vi "main.vi"() -> ()   [LabVIEW 2013]
uses:
  <vilib>/Utility/file.llb/Read From Spreadsheet File (DBL).vi
panel:
  out "Current file num":i32
  out "ROI Width":u32
  out "ROI Height":u32
  in  "Image Dark":dbl[][](array[numeric])
  in  "Image Light":dbl[][](array[numeric])
  in  "Image Atom":dbl[][](array[numeric])
  out "Best fit parameters":dbl[](array[numeric])
  out "Fitting Results Save Path":string[](array[string])
  out "Best fit results":dbl[][](array[numeric])
  in  "Initial guess values":dbl[](array[numeric])
  in  "Latest image data":dbl[][](array[numeric])
  out "Fitting Type":u16(ring)
  out "Force Guess?":bool
  out "Aquired?":bool
  out "Process Index":i32
  out "External Trigger":bool
  out "XY图":cluster{dbl[], dbl[]}[](graph)
  out "OD Image":dbl[][](graph)
  in  "OD fit":bool
  in  "OD num":i32
  out "Fit Done":bool
  in  "Exit":bool
  out "XY图 2":cluster{dbl[], dbl[]}[](graph)
  in  "Auto Split":bool
  in  "Fit":bool
  in  "Open File":bool
  in  "Auto Fit":bool
  in  "Stop":bool
  in  "Aquire":bool
  in  "Fitting Config":bool
  in  "Camera Config":bool
  in  "Initialize":bool
  in  "Live Image Display":refnum<k7>(container)
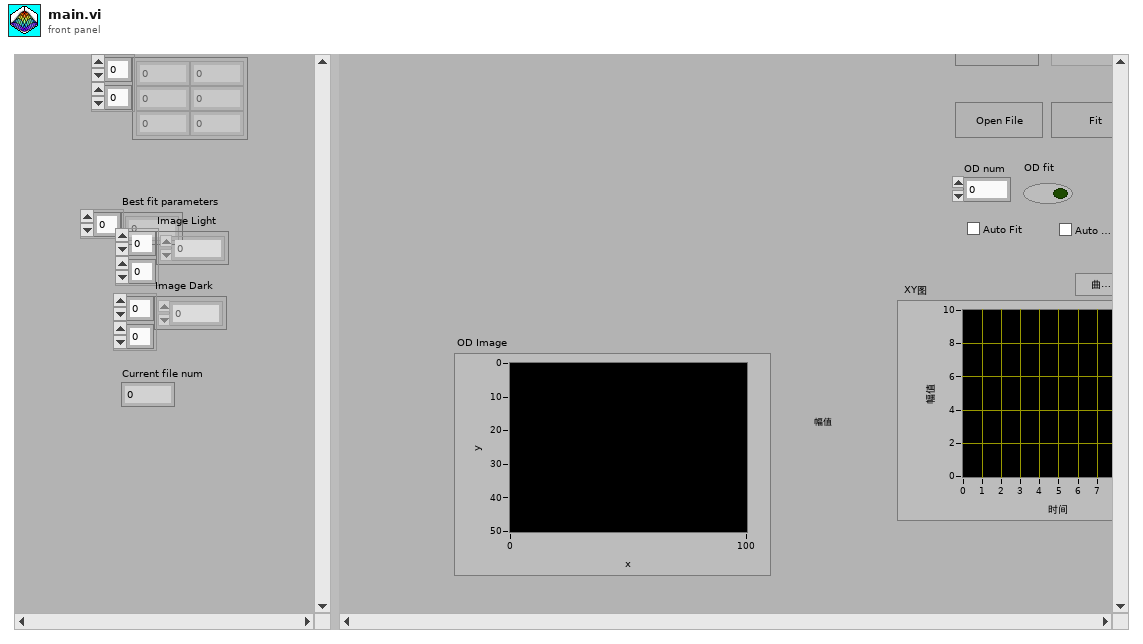
[diagram p1: front panel]
types:
  T1 = enum8{"Enabled", "Disabled", "Disabled and Grayed Out"}
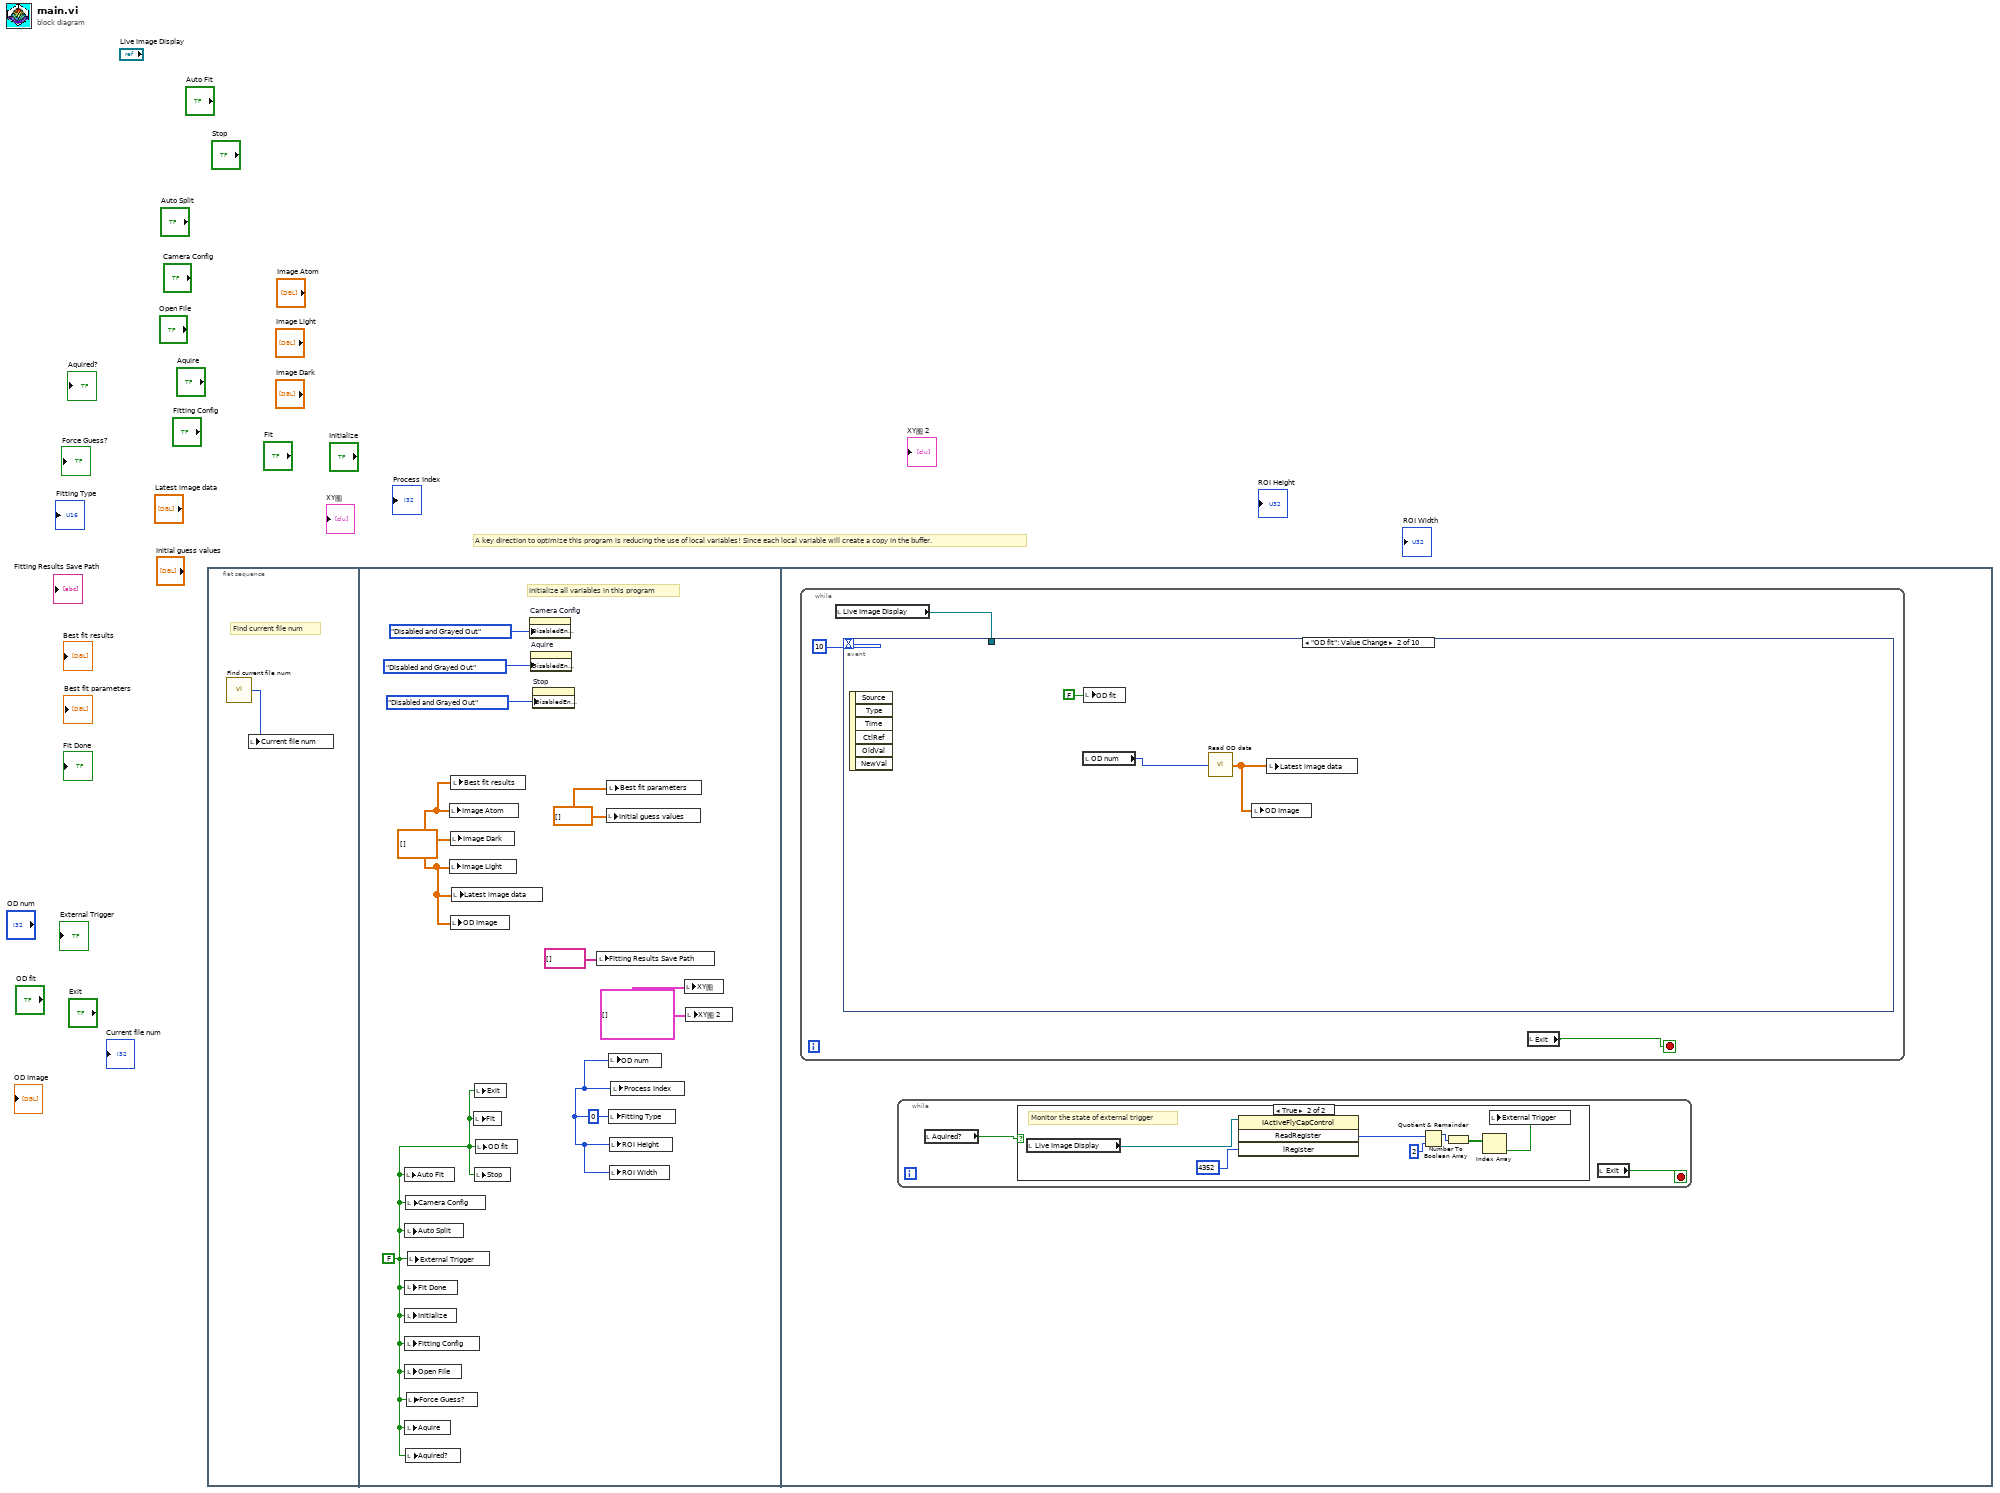
[diagram p0: block diagram]
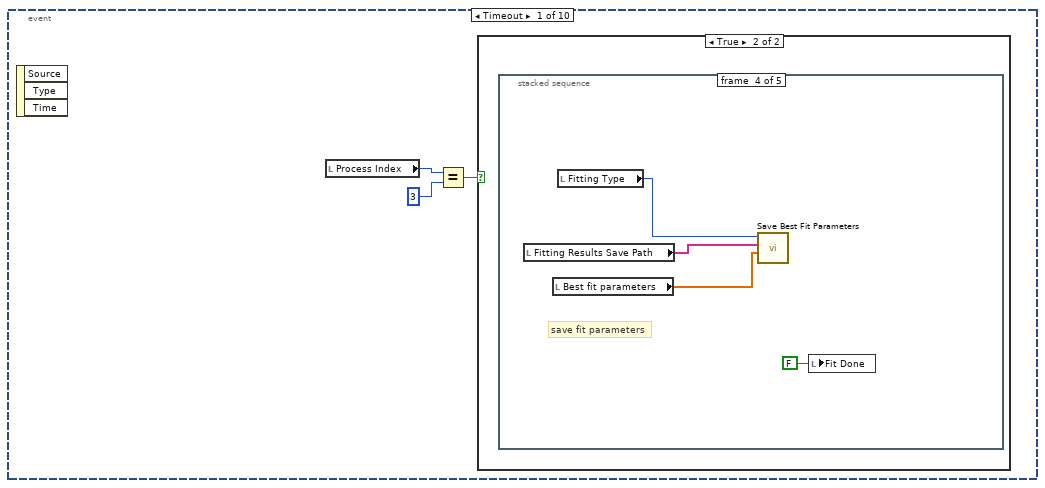
[diagram p3: hidden frame]
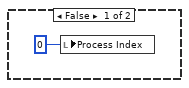
[diagram p4: hidden frame]
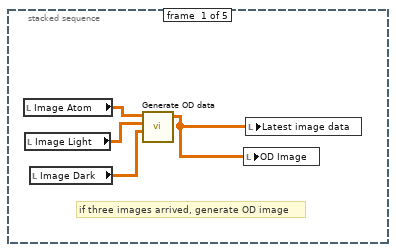
[diagram p5: hidden frame]
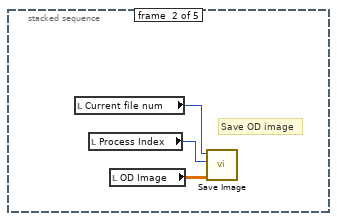
[diagram p6: hidden frame]
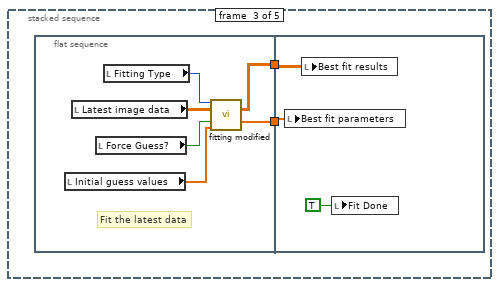
[diagram p7: hidden frame]
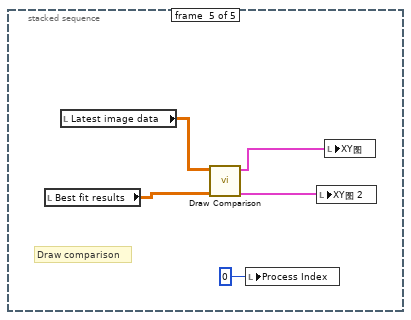
[diagram p8: hidden frame]
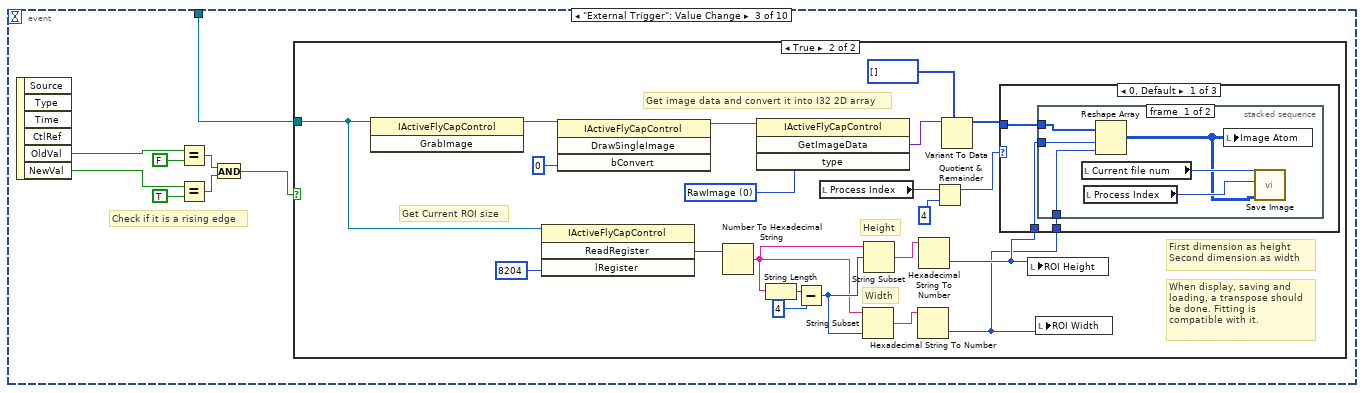
[diagram p9: hidden frame]
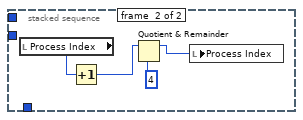
[diagram p11: hidden frame]
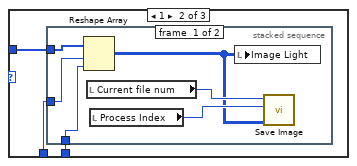
[diagram p12: hidden frame]
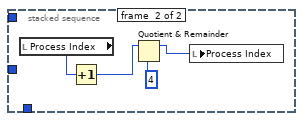
[diagram p13: hidden frame]
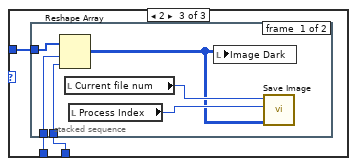
[diagram p14: hidden frame]
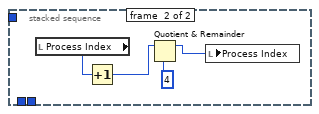
[diagram p15: hidden frame]
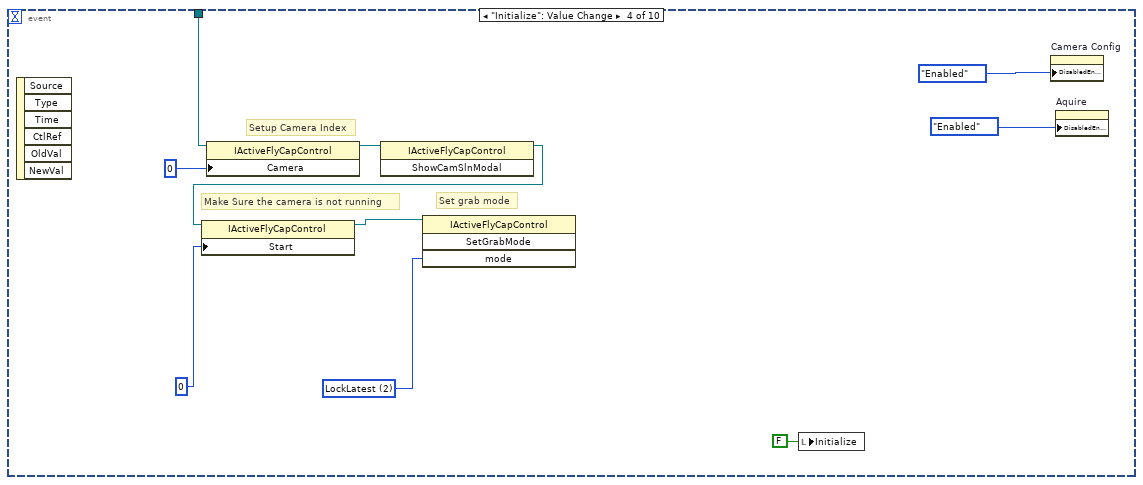
[diagram p16: hidden frame]
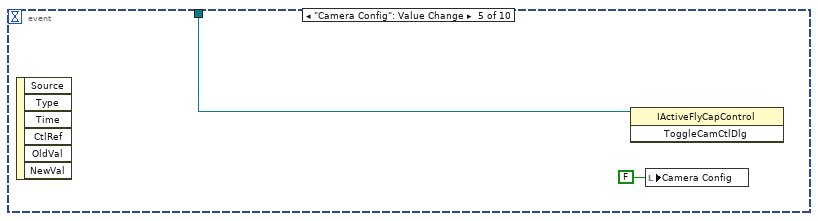
[diagram p17: hidden frame]
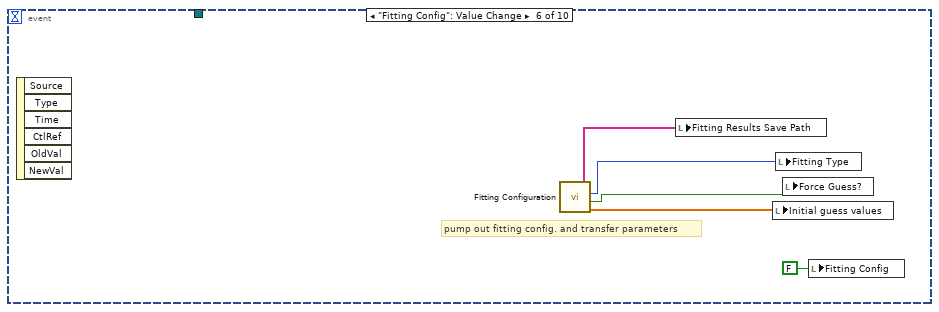
[diagram p18: hidden frame]
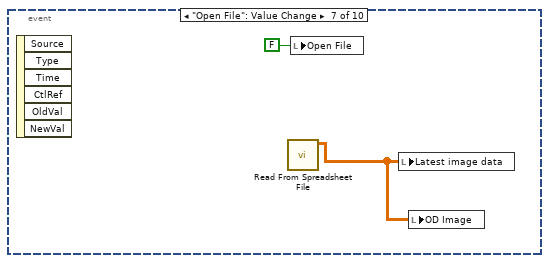
[diagram p19: hidden frame]
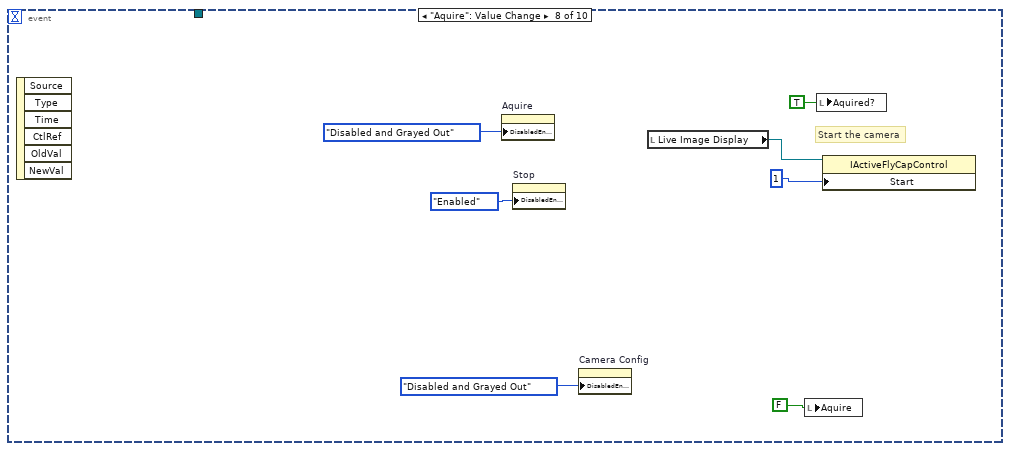
[diagram p20: hidden frame]
diagram:
  # "A key direction to optimize this program is reducing the use of local variables! Since each local variable will create a copy in the buffer."
  n1 = flat-sequence {
    frame #0 {
      # "Find current file num"
      n2 = call "Find current file num.vi"() -> ("Current File Num"=w1:u16)  [unwired: 2 in]
      n3 = local write "Current file num"(w1) -> ()
    }
    frame #1 {
      w4 = cluster{dbl[], dbl[]}[] [] ("XY图")
      w3 = 0 ("OD num")
      w7 = dbl[][] [] ("Best fit results")
      w6 = dbl[] [] ("Best fit parameters")
      w2 = FALSE ("Aquire")
      # "Initialize all variables in this program"
      n4 = local write "Auto Fit"(w2) -> ()
      n5 = local write "Auto Split"(w2) -> ()
      n6 = local write "Fit Done"(w2) -> ()
      n7 = local write "Initialize"(w2) -> ()
      n8 = local write "Fitting Config"(w2) -> ()
      n9 = local write "Open File"(w2) -> ()
      n10 = local write "Aquire"(w2) -> ()
      n11 = local write "Camera Config"(w2) -> ()
      n12 = local write "Aquired?"(w2) -> ()
      n13 = local write "Force Guess?"(w2) -> ()
      n14 = local write "External Trigger"(w2) -> ()
      n15 = local write "Image Atom"(w7) -> ()
      n16 = local write "Image Light"(w7) -> ()
      n17 = local write "Image Dark"(w7) -> ()
      n18 = local write "OD Image"(w7) -> ()
      n19 = local write "Best fit results"(w7) -> ()
      n20 = local write "Latest image data"(w7) -> ()
      n21 = local write "Fit"(w2) -> ()
      n22 = local write "Exit"(w2) -> ()
      n23 = local write "Stop"(w2) -> ()
      n24 = local write "OD fit"(w2) -> ()
      n25 = property on="Camera Config" class="Bool (strict)"("DisabledEnum"=T1."Disabled and Grayed Out" ("禁用")) -> ()  [unwired: 2 in, 2 out]
      n26 = property on="Aquire" class="Bool (strict)"("DisabledEnum"=T1."Disabled and Grayed Out" ("禁用")) -> ()  [unwired: 2 in, 2 out]
      n27 = property on="Stop" class="Bool (strict)"("DisabledEnum"=T1."Disabled and Grayed Out" ("禁用")) -> ()  [unwired: 2 in, 2 out]
      n28 = local write "Fitting Results Save Path"(string[] [] ("Fitting Results Save Path")) -> ()
      n29 = local write "Initial guess values"(w6) -> ()
      n30 = local write "Best fit parameters"(w6) -> ()
      n31 = local write "OD num"(w3) -> ()
      n32 = local write "Fitting Type"(w3) -> ()
      n33 = local write "ROI Height"(w3) -> ()
      n34 = local write "ROI Width"(w3) -> ()
      n35 = local write "Process Index"(w3) -> ()
      n36 = local write "XY图"(w4) -> ()
      n37 = local write "XY图 2"(w4) -> ()
    }
    frame #2 {
      n38 = while {
        stop <- w20 stop-if-true
        n39 = local read "Live Image Display"() -> (w21:refnum<k7>)
        n40 = event shown="[1] \"OD fit\": Value Change" {
          selector: _ -> [_ _ _ _ _ _ _ _ _ _]
          dyn-events: _ -> [_ _ _ _ _ _ _ _ _ _]
          timeout: 10 -> [_ _ _ _ _ _ _ _ _ _]
          tunnel: w21 -> [_ _ w57 w128 w136 _ _ _ _ _]
          event Timeout {
            n41 = event-data() -> ()  [unwired: 1 in, 3 out]
            n42 = local read "Process Index"() -> (w25:i32)
            n43 = Equal?(x=w25, y=3) -> (x = y?=w23:bool)
            n44 = case shown="True" w23 {
              frame False {
                n45 = local write "Process Index"(0 ("Process Index")) -> ()
              }
              frame True {
                n46 = stacked-sequence {
                  frame #0 {
                    # "if three images arrived, generate OD image"
                    n47 = local read "Image Atom"() -> (w30:dbl[][])
                    n48 = local read "Image Light"() -> (w29:dbl[][])
                    n49 = local read "Image Dark"() -> (w28:dbl[][])
                    n50 = call "Generate OD data.vi"("dark"=w28, "light"=w29, "atom"=w30) -> ("OD image"=w27:dbl[][])  [unwired: 3 in]
                    n51 = local write "OD Image"(w27) -> ()
                    n52 = local write "Latest image data"(w27) -> ()
                  }
                  frame #1 {
                    # "Save OD image"
                    n53 = local read "Current file num"() -> (w33:i32)
                    n54 = local read "Process Index"() -> (w32:i32)
                    n55 = local read "OD Image"() -> (w31:dbl[][])
                    n56 = call "Save Image.vi"("Data"=w31, "Process Index"=w32, "Current File Num"=w33) -> ()  [unwired: 9 in]
                  }
                  frame #2 {
                    n57 = flat-sequence {
                      tunnel: [w37] -> w35
                      tunnel: [w36] -> w34
                      tunnel: w35 -> [w44]
                      tunnel: w34 -> [w43]
                      frame #0 {
                        # "Fit the latest data"
                        n58 = local read "Initial guess values"() -> (w38:dbl[])
                        n59 = local read "Latest image data"() -> (w40:dbl[][])
                        n60 = local read "Force Guess?"() -> (w39:bool)
                        n61 = local read "Fitting Type"() -> (w41:u16)
                        n62 = call "fitting modified.vi"("fitting type"=w41, "2D data"=w40, "force guess?"=w39, "intial guess value"=w38) -> ("best fit"=w37:dbl[][], "best fit parameters"=w36:dbl[])  [unwired: 9 in, 1 out]
                      }
                      frame #1 {
                        n63 = local write "Best fit parameters"(w43) -> ()
                        n64 = local write "Best fit results"(w44) -> ()
                        n65 = local write "Fit Done"(TRUE ("Fit Done")) -> ()
                      }
                    }
                  }
                  frame #3 {
                    # "save fit parameters"
                    n66 = local read "Fitting Results Save Path"() -> (w47:string[])
                    n67 = local read "Best fit parameters"() -> (w46:dbl[])
                    n68 = local read "Fitting Type"() -> (w48:u16)
                    n69 = call "Save Best Fit Parameters.vi"("Best Fit Parameters"=w46, "Fitting Results Save Path"=w47, "Fitting Type"=w48) -> ()  [unwired: 9 in]
                    n70 = local write "Fit Done"(FALSE ("Fit Done")) -> ()
                  }
                  frame #4 {
                    # "Draw comparison"
                    n71 = local read "Best fit results"() -> (w51:dbl[][])
                    n72 = local read "Latest image data"() -> (w50:dbl[][])
                    n73 = call "Draw Comparison.vi"("Best Fit"=w51, "Raw Data"=w50) -> ("Vertical Comparison"=w52:cluster{i32[], dbl[]}[], "Horizontal Comparison"=w53:cluster{i32[], dbl[]}[])  [unwired: 7 in]
                    n74 = local write "Process Index"(0 ("Process Index")) -> ()
                    n75 = local write "XY图 2"(w52) -> ()
                    n76 = local write "XY图"(w53) -> ()
                  }
                }
              }
            }
          }
          event "OD fit": Value Change {
            n77 = event-data() -> ()  [unwired: 1 in, 6 out]
            n78 = local read "OD num"() -> (w55:i32)
            n79 = local write "OD fit"(FALSE ("OD fit")) -> ()
            n80 = call "Read OD data.vi"("OD num"=w55) -> ("OD data"=w54:dbl[][])  [unwired: 4 in]
            n81 = local write "OD Image"(w54) -> ()
            n82 = local write "Latest image data"(w54) -> ()
          }
          event "External Trigger": Value Change {
            # "Check if it is a rising edge"
            n83 = event-data() -> ("OldVal"=w62:bool, "NewVal"=w61:bool)  [unwired: 1 in, 4 out]
            n84 = Equal?(x=w62, y=FALSE) -> (x = y?=w64:bool)
            n85 = Equal?(x=w61, y=TRUE) -> (x = y?=w63:bool)
            n86 = And(x=w64, y=w63) -> (x .and. y?=w58:bool)
            n87 = case shown="True" w58 {
              tunnel: w57 -> [_ w81]
              frame False {
              }
              frame True {
                w82 = 0 items=["RawImage", "ColorProcessedImage"] ("type")
                # "Get image data and convert it into I32 2D array"
                # "When display, saving and \nloading, a transpose should\nbe done. Fitting is \ncompatible with it."
                # "First dimension as height\nSecond dimension as width"
                # "Width"
                # "Height"
                # "Get Current ROI size"
                n88 = invoke class="IActiveFlyCapControl" method="GrabImage"(reference=w81) -> (reference out=w85:refnum<k7>)  [unwired: 2 in, 2 out]
                n89 = invoke class="IActiveFlyCapControl" method="ReadRegister"(reference=w81, "lRegister"=u32 8204) -> ("ReadRegister"=w78:u32)  [unwired: 2 in, 3 out]
                n90 = invoke class="IActiveFlyCapControl" method="DrawSingleImage"(reference=w85, "bConvert"=0) -> (reference out=w84:refnum<k7>)  [unwired: 2 in, 3 out]
                n91 = Number To Hexadecimal String(2:w78) -> (0:w74:string)  [unwired: 1 in]
                n92 = invoke class="IActiveFlyCapControl" method="GetImageData"(reference=w84, "type"=w82) -> ("GetImageData"=w79:variant)  [unwired: 2 in, 3 out]
                n93 = String Length(string=w74) -> (length=w77:i32)
                n94 = Subtract(x=w77, y=4) -> (x-y=w75:i32)
                n95 = local read "Process Index"() -> (w70:i32)
                n96 = String Subset(string=w74, length (rest)=w75) -> (substring=w71:string)  [unwired: 1 in]
                n97 = String Subset(string=w74, offset (0)=w75) -> (substring=w72:string)  [unwired: 1 in]
                n98 = Hexadecimal String To Number(string=w71) -> (number=w65:u32)  [unwired: 2 in, 1 out]
                n99 = Hexadecimal String To Number(string=w72) -> (number=w66:u32)  [unwired: 2 in, 1 out]
                n100 = Quotient & Remainder(x=w70, y=4) -> (x-y*floor(x/y)=w68:i32)  [unwired: 1 out]
                n101 = Variant To Data(type=i32[] [], Variant=w79) -> (data=w67:i32[])  [unwired: 1 in, 1 out]
                n102 = case shown="0, Default" w68 {
                  tunnel: w67 -> [w88 w101 w114]
                  tunnel: w66 -> [w87 w100 w113]
                  tunnel: w65 -> [w86 w99 w112]
                  frame 0, Default {
                    n103 = stacked-sequence {
                      tunnel: w88 -> [w92 _]
                      tunnel: w87 -> [w91 _]
                      tunnel: w86 -> [w90 _]
                      frame #0 {
                        n104 = local read "Current file num"() -> (w94:i32)
                        n105 = local read "Process Index"() -> (w93:i32)
                        n106 = Reshape Array(w92, w91, w90) -> (w89:i32[][])
                        n107 = local write "Image Atom"(w89) -> ()
                        n108 = call "Save Image.vi"("Data"=w89, "Process Index"=w93, "Current File Num"=w94) -> ()  [unwired: 9 in]
                      }
                      frame #1 {
                        n109 = local read "Process Index"() -> (w98:i32)
                        n110 = Increment(x=w98) -> (x+1=w97:i32)
                        n111 = Quotient & Remainder(x=w97, y=4) -> (x-y*floor(x/y)=w95:i32)  [unwired: 1 out]
                        n112 = local write "Process Index"(w95) -> ()
                      }
                    }
                  }
                  frame 1 {
                    n113 = stacked-sequence {
                      tunnel: w101 -> [w103 _]
                      tunnel: w100 -> [w105 _]
                      tunnel: w99 -> [w104 _]
                      frame #0 {
                        n114 = Reshape Array(w103, w105, w104) -> (w102:i32[][])
                        n115 = local read "Current file num"() -> (w107:i32)
                        n116 = local read "Process Index"() -> (w106:i32)
                        n117 = local write "Image Light"(w102) -> ()
                        n118 = call "Save Image.vi"("Data"=w102, "Process Index"=w106, "Current File Num"=w107) -> ()  [unwired: 9 in]
                      }
                      frame #1 {
                        n119 = local read "Process Index"() -> (w111:i32)
                        n120 = Increment(x=w111) -> (x+1=w110:i32)
                        n121 = Quotient & Remainder(x=w110, y=4) -> (x-y*floor(x/y)=w108:i32)  [unwired: 1 out]
                        n122 = local write "Process Index"(w108) -> ()
                      }
                    }
                  }
                  frame 2 {
                    n123 = stacked-sequence {
                      tunnel: w114 -> [w118 _]
                      tunnel: w113 -> [w117 _]
                      tunnel: w112 -> [w116 _]
                      frame #0 {
                        n124 = Reshape Array(w118, w117, w116) -> (w115:i32[][])
                        n125 = local read "Current file num"() -> (w120:i32)
                        n126 = local read "Process Index"() -> (w119:i32)
                        n127 = local write "Image Dark"(w115) -> ()
                        n128 = call "Save Image.vi"("Data"=w115, "Process Index"=w119, "Current File Num"=w120) -> ()  [unwired: 9 in]
                      }
                      frame #1 {
                        n129 = local read "Process Index"() -> (w124:i32)
                        n130 = Increment(x=w124) -> (x+1=w123:i32)
                        n131 = Quotient & Remainder(x=w123, y=4) -> (x-y*floor(x/y)=w121:i32)  [unwired: 1 out]
                        n132 = local write "Process Index"(w121) -> ()
                      }
                    }
                  }
                }
                n133 = local write "ROI Height"(w66) -> ()
                n134 = local write "ROI Width"(w65) -> ()
              }
            }
          }
          event "Initialize": Value Change {
            w132 = 2 items=["FreeRunning", "LockNext", "LockLatest"] ("mode")
            # "Setup Camera Index"
            # "Set grab mode"
            # "Make Sure the camera is not running"
            n135 = event-data() -> ()  [unwired: 1 in, 6 out]
            n136 = property class="IActiveFlyCapControl"(reference=w128, "Camera"=0 ("Start")) -> (reference out=w131:refnum<k7>)  [unwired: 1 in, 1 out]
            n137 = invoke class="IActiveFlyCapControl" method="ShowCamSlnModal"(reference=w131) -> (reference out=w127:refnum<k7>)  [unwired: 2 in, 2 out]
            n138 = property class="IActiveFlyCapControl"(reference=w127, "Start"=0 ("Camera")) -> (reference out=w126:refnum<k7>)  [unwired: 1 in, 1 out]
            n139 = invoke class="IActiveFlyCapControl" method="SetGrabMode"(reference=w126, "mode"=w132) -> ()  [unwired: 2 in, 4 out]
            n140 = local write "Initialize"(FALSE ("Initialize")) -> ()
            n141 = property on="Camera Config" class="Bool (strict)"("DisabledEnum"=T1."Enabled" ("禁用")) -> ()  [unwired: 2 in, 2 out]
            n142 = property on="Aquire" class="Bool (strict)"("DisabledEnum"=T1."Enabled" ("禁用")) -> ()  [unwired: 2 in, 2 out]
          }
          event "Camera Config": Value Change {
            n143 = event-data() -> ()  [unwired: 1 in, 6 out]
            n144 = invoke class="IActiveFlyCapControl" method="ToggleCamCtlDlg"(reference=w136) -> ()  [unwired: 2 in, 3 out]
            n145 = local write "Camera Config"(FALSE ("Camera Config")) -> ()
          }
          event "Fitting Config": Value Change {
            # "pump out fitting config. and transfer parameters"
            n146 = event-data() -> ()  [unwired: 1 in, 6 out]
            n147 = call "Fitting Configuration.vi"() -> ("intial guess"=w140:dbl[], "Force Guess？"=w139:bool, "Fitting Type"=w138:u16, "Fitting Results Save Path"=w137:string[])  [unwired: 5 in]
            n148 = local write "Fitting Results Save Path"(w137) -> ()
            n149 = local write "Initial guess values"(w140) -> ()
            n150 = local write "Fitting Type"(w138) -> ()
            n151 = local write "Force Guess?"(w139) -> ()
            n152 = local write "Fitting Config"(FALSE ("Fitting Config")) -> ()
          }
          event "Open File": Value Change {
            n153 = event-data() -> ()  [unwired: 1 in, 6 out]
            n154 = call-poly <vilib>:"Read From Spreadsheet File.vi"() -> ("all rows"=w142:dbl[][])  [unwired: 7 in, 4 out]
            n155 = local write "Open File"(FALSE ("Open File")) -> ()
            n156 = local write "Latest image data"(w142) -> ()
            n157 = local write "OD Image"(w142) -> ()
          }
          event "Aquire": Value Change {
            # "Start the camera"
            n158 = event-data() -> ()  [unwired: 1 in, 6 out]
            n159 = property on="Aquire" class="Bool (strict)"("DisabledEnum"=T1."Disabled and Grayed Out" ("禁用")) -> ()  [unwired: 2 in, 2 out]
            n160 = property on="Stop" class="Bool (strict)"("DisabledEnum"=T1."Enabled" ("禁用")) -> ()  [unwired: 2 in, 2 out]
            n161 = property on="Camera Config" class="Bool (strict)"("DisabledEnum"=T1."Disabled and Grayed Out" ("禁用")) -> ()  [unwired: 2 in, 2 out]
            n162 = local read "Live Image Display"() -> (w145:refnum<k7>)
            n163 = local write "Aquire"(FALSE ("Initialize")) -> ()
            n164 = local write "Aquired?"(TRUE ("Aquired?")) -> ()
            n165 = property class="IActiveFlyCapControl"(reference=w145, "Start"=1) -> ()  [unwired: 1 in, 2 out]
          }
          event "Stop": Value Change {
            # "stop the camera"
            n166 = event-data() -> ()  [unwired: 1 in, 6 out]
            n167 = local read "Live Image Display"() -> (w153:refnum<k7>)
            n168 = local write "Stop"(FALSE ("Initialize")) -> ()
            n169 = property on="Stop" class="Bool (strict)"("DisabledEnum"=T1."Disabled and Grayed Out" ("禁用")) -> ()  [unwired: 2 in, 2 out]
            n170 = property on="Aquire" class="Bool (strict)"("DisabledEnum"=T1."Disabled and Grayed Out" ("禁用")) -> ()  [unwired: 2 in, 2 out]
            n171 = property class="IActiveFlyCapControl"(reference=w153, "Start"=0) -> (reference out=w152:refnum<k7>)  [unwired: 1 in, 1 out]
            n172 = local write "Aquired?"(FALSE ("Aquired?")) -> ()
            n173 = local write "Live Image Display"(w152) -> ()
          }
          event "Fit": Value Change {
            n174 = event-data() -> ()  [unwired: 1 in, 6 out]
            n175 = stacked-sequence {
              frame #0 {
                n176 = flat-sequence {
                  tunnel: [w161] -> w159
                  tunnel: [w160] -> w158
                  tunnel: w159 -> [w169]
                  tunnel: w158 -> [w168]
                  frame #0 {
                    # "Fit the latest data"
                    n177 = local read "Initial guess values"() -> (w164:dbl[])
                    n178 = local read "Latest image data"() -> (w163:dbl[][])
                    n179 = local read "Force Guess?"() -> (w165:bool)
                    n180 = local read "Fitting Type"() -> (w162:u16)
                    n181 = call "fitting modified.vi"("fitting type"=w162, "2D data"=w163, "force guess?"=w165, "intial guess value"=w164) -> ("best fit"=w161:dbl[][], "best fit parameters"=w160:dbl[])  [unwired: 9 in, 1 out]
                  }
                  frame #1 {
                    n182 = local write "Fit"(FALSE ("Fit")) -> ()
                    n183 = local write "Best fit results"(w169) -> ()
                    n184 = local write "Best fit parameters"(w168) -> ()
                    n185 = local write "Fit Done"(TRUE ("Fit Done")) -> ()
                  }
                }
              }
              frame #1 {
                # "Save best fit parameters"
                n186 = local read "Fitting Results Save Path"() -> (w171:string[])
                n187 = local read "Best fit parameters"() -> (w170:dbl[])
                n188 = local read "Fitting Type"() -> (w172:u16)
                n189 = call "Save Best Fit Parameters.vi"("Best Fit Parameters"=w170, "Fitting Results Save Path"=w171, "Fitting Type"=w172) -> ()  [unwired: 9 in]
                n190 = local write "Fit Done"(FALSE ("Fit Done")) -> ()
              }
              frame #2 {
                # "Draw Comparison"
                n191 = local read "Latest image data"() -> (w178:dbl[][])
                n192 = local read "Best fit results"() -> (w177:dbl[][])
                n193 = call "Draw Comparison.vi"("Best Fit"=w177, "Raw Data"=w178) -> ("Vertical Comparison"=w175:cluster{i32[], dbl[]}[], "Horizontal Comparison"=w176:cluster{i32[], dbl[]}[])  [unwired: 7 in]
                n194 = local write "Fit"(FALSE ("Initialize")) -> ()
                n195 = local write "XY图 2"(w175) -> ()
                n196 = local write "XY图"(w176) -> ()
              }
            }
          }
        }
        n197 = local read "Exit"() -> (w20:bool)
      }
      n198 = while {
        stop <- w12 stop-if-true
        n199 = local read "Aquired?"() -> (w11:bool)
        n200 = case shown="True" w11 {
          frame False {
          }
          frame True {
            # "Monitor the state of external trigger"
            n201 = local read "Live Image Display"() -> (w19:refnum<k7>)
            n202 = invoke class="IActiveFlyCapControl" method="ReadRegister"(reference=w19, "lRegister"=u32 4352) -> ("ReadRegister"=w17:u32)  [unwired: 2 in, 3 out]
            n203 = Quotient & Remainder(x=w17, y=u32 2) -> (x-y*floor(x/y)=w15:u32)  [unwired: 1 out]
            n204 = Number To Boolean Array(number=w15) -> (Boolean array=w14:bool[])
            n205 = Index Array(array=w14) -> (element=w13:bool)  [unwired: 1 in]
            n206 = local write "External Trigger"(w13) -> ()
          }
        }
        n207 = local read "Exit"() -> (w12:bool)
      }
    }
  }
